vi "PCO_ClearRamSegment.vi"(8 "error in (no error)":errorcluster {"code" format="%x"}, 11 "ph":u64) -> (0 "error out":errorcluster {"code" format="%x"}, 2 "ErrorMessage":i32 format="%x", 3 "ph out":u64)   [LabVIEW 2019, in "SDK.lvlib" / "StorageControl.lvlib"]
doc: "<b>Description:</b>\nThis function does clear the active memory segment. All image data is cleared and the segment is prepared for new images.\n\n<b>Supported camera type:</b>\npco.dimax, pco.1200, pco.1600, pco.2000, pco.4000\n\n<b>Descriptor dependency:</b>\ndwGeneralCapsDESC1: NO_RECORDER"
uses:
  StorageControl.lvlib
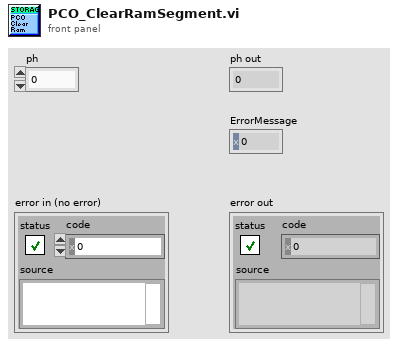
[diagram p1: front panel]
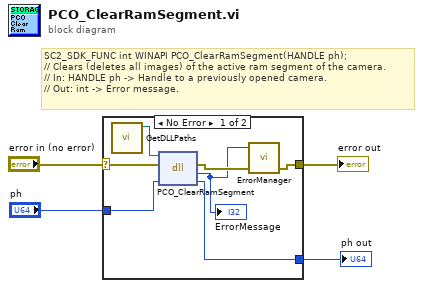
[diagram p0: block diagram]
diagram:
  # "SC2_SDK_FUNC int WINAPI PCO_ClearRamSegment(HANDLE ph);\n// Clears (deletes all images) of the active ram segment of the camera.\n// In: HANDLE ph -> Handle to a previously opened camera.\n// Out: int -> Error message."
  n1 = case shown="No Error" "error in (no error)" {
    selector: "error in (no error)" -> [w9 w13]
    tunnel: "ph" -> [w11 w12]
    tunnel: [w10 w12] -> w3
    tunnel: [w7 w13] -> w2
    frame No Error {
      n2 = call "GetDLLPaths.vi"() -> ("SC2_Cam_Path"=w5:path)  [unwired: 8 in, 3 out]
      n3 = dll-call lib="?" fn="PCO_ClearRamSegment"(path in=w5, error in=w9, "ph"=w11) -> (error out=w8:errorcluster, "return type"=w6:i32, "ph"=w10:u64)  [unwired: 1 in, 1 out]
      "ErrorMessage" <- w6
      n4 = call "ErrorManager.vi"("error in (no error)"=w8, "error code"=w6) -> ("error out"=w7:errorcluster)  [unwired: 2 in, 1 out]
    }
    frame Error {
    }
  }
  "ph out" <- w3
  "error out" <- w2
